vi "Huffman Compression.vi"() -> ()   [LabVIEW 2017]
uses:
  BinaryNode.ctl
panel:
  out "Compression ratio":dbl
  out "Letters & their occurences":string[][](array[string])
  out "Size after compression (bits)":i32
  out "Compressed text":string
  out "Size before compression (bits)":i32
  out "Table of Huffman Codes":string[][](array[string])
  out "Linked List":T1[](array[typedef])
  in  "Text to compress":string="a woodchuck should chuck if a woodchuck could chuck wood as long as a woodchuck would chuck wood"
  # "Overview: Demonstrates how to create Huffman codes for text compression.\nRequirements: LabVIEW Full Development System 2017 or compatible\nInstructions:\n1. Enter a text to compress in the \"Text to compress\" box.\n2. Run this Vi.\n3. Open the block diagram and sub-Vis for comments.\n\nThis program is not the ideal, quickest solution to get Huffman coding but is made as a demonstration. The coding is made at a letter level.\n\nSources:\nhttps://en.wikipedia.org/wiki/Huffman_coding\nhttps://people.ok.ubc.ca/ylucet/DS/Huffman.html"
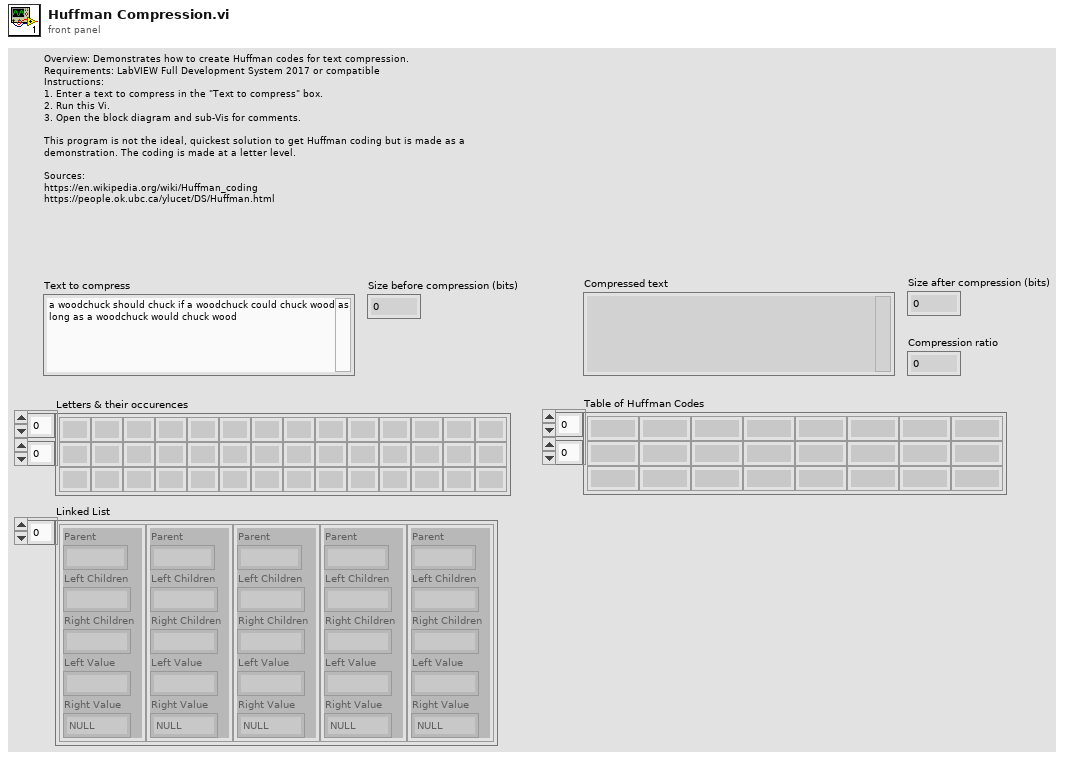
[diagram p1: front panel]
types:
  T1 = typedef "BinaryNode.ctl" = cluster{"Parent":string, "Left Children":string, "Right Children":string, "Left Value":string, "Right Value":string}
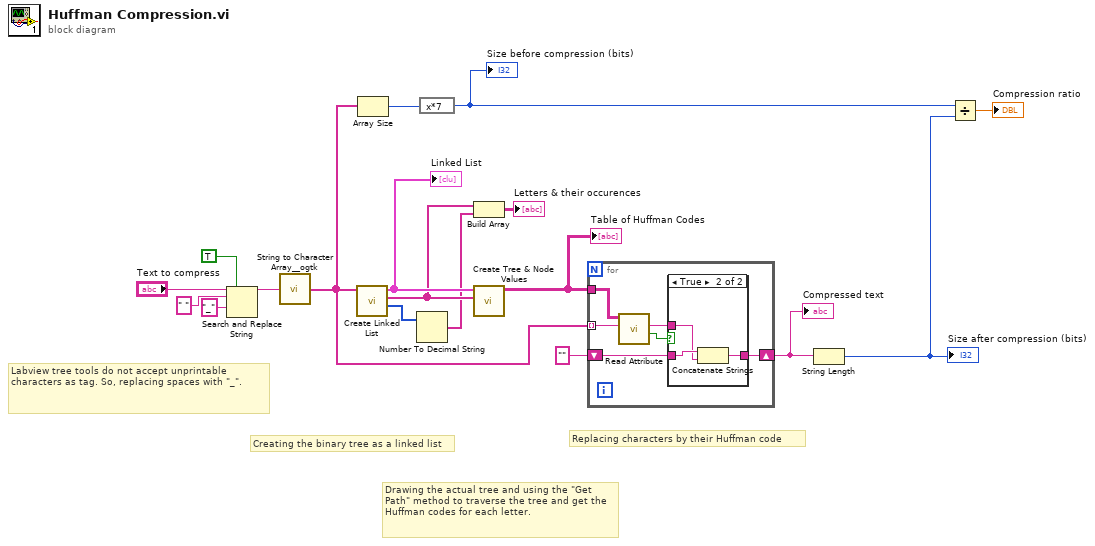
[diagram p0: block diagram]
diagram:
  # "Replacing characters by their Huffman code"
  # "Drawing the actual tree and using the \"Get Path\" method to traverse the tree and get the Huffman codes for each letter."
  # "Creating the binary tree as a linked list"
  # "Labview tree tools do not accept unprintable characters as tag. So, replacing spaces with \"_\"."
  n1 = Search and Replace String(replace all?=TRUE ("replace all? (F)"), input string="Text to compress", search string=" ", replace string="_" ("replace string (\"\")")) -> (result string=w4:string)  [unwired: 4 in, 3 out]
  n2 = call <userlib>:"String to Character Array__ogtk.vi"("Input String"=w4) -> ("Character Array"=w6:string[])
  n3 = call "Create Linked List.vi"("Text array to compress"=w6) -> ("Sorted Occurences"=w13:i32[], "Sorted Letters"=w12:string[], "Linked Nodes OUT"=w14:T1[])  [unwired: 8 in]
  "Linked List" <- w14
  n4 = Array Size(array=w6) -> (size(s)=w18:i32)
  n5 = Number To Decimal String(number=w13) -> (decimal integer string=w11:string[])  [unwired: 1 in]
  n6 = expression code="x*7"(w18) -> (w9:i32)
  "Size before compression (bits)" <- w9
  n7 = Build Array(w12, w11) -> (→"Letters & their occurences":string[][])
  n8 = call "Create Tree & Node Values.vi"("Letters to code"=w12, "Linked Nodes IN"=w14) -> ("Huffman codes for each letter"=w15:string[][])  [unwired: 8 in, 1 out]
  "Table of Huffman Codes" <- w15
  n9 = for {
    tunnel: w6 -> [w21] mode=indexing
    shift-right: [w23] -> w16
    shift-left: "" -> [w24]
    tunnel: w15 -> [w22]
    n10 = call "Read Attribute.vi"("Attribute to Read"=w21, "Object Attributes IN"=w22) -> ("Found?"=w20:bool, "Attribute Value"=w19:string)  [unwired: 7 in, 1 out]
    n11 = case shown="True" w20 {
      tunnel: w24 -> [w25 w28]
      tunnel: [w25 w27] -> w23
      tunnel: w19 -> [_ w26]
      frame False {
      }
      frame True {
        n12 = Concatenate Strings(w28, w26) -> (w27:string)
      }
    }
  }
  "Compressed text" <- w16
  n13 = String Length(string=w16) -> (length=w8:i32)
  "Size after compression (bits)" <- w8
  n14 = Divide(x=w9, y=w8) -> (x/y=→"Compression ratio":dbl)
